vi "take img.vi"() -> ()   [LabVIEW 2019]
uses:
  <vilib>/userDefined/High Color/IMAQdx.ctl
  <vilib>/vision/driver/NI_Vision_Acquisition_Software.lvlib
panel:
  out "error out":errorcluster
  in  "stop":bool
  in  "Boolean":bool
  out "Image":T1(plugin-control)
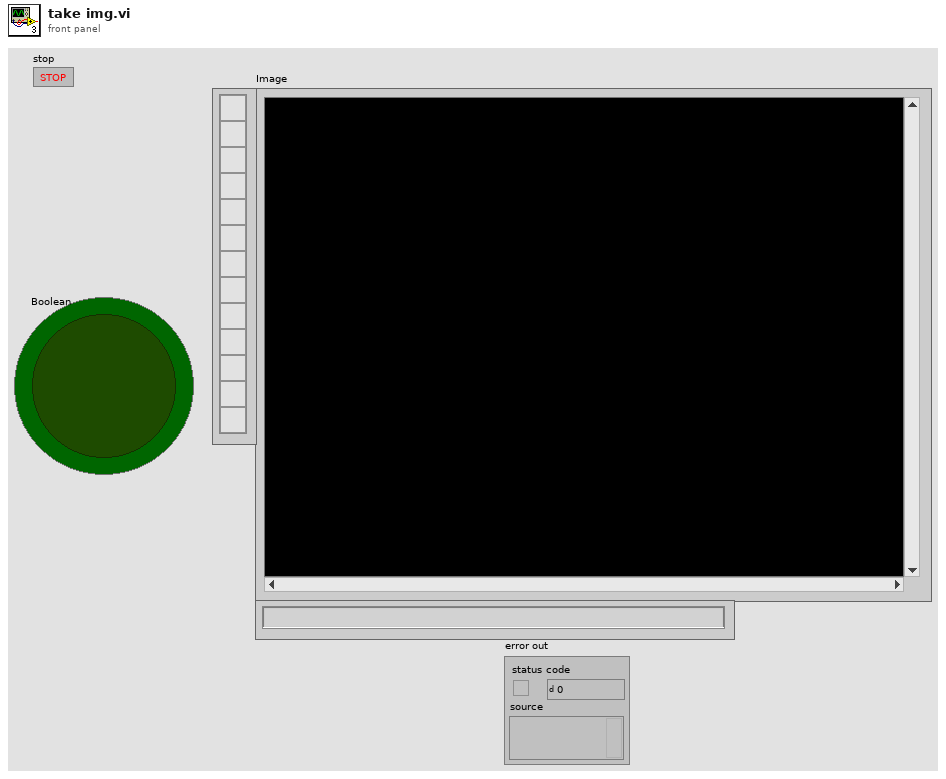
[diagram p1: front panel]
types:
  T1 = typedef "IMAQ Image.ctl" = refnum<image>
  T2 = typedef "IMAQdx.ctl" = refnum<k21>
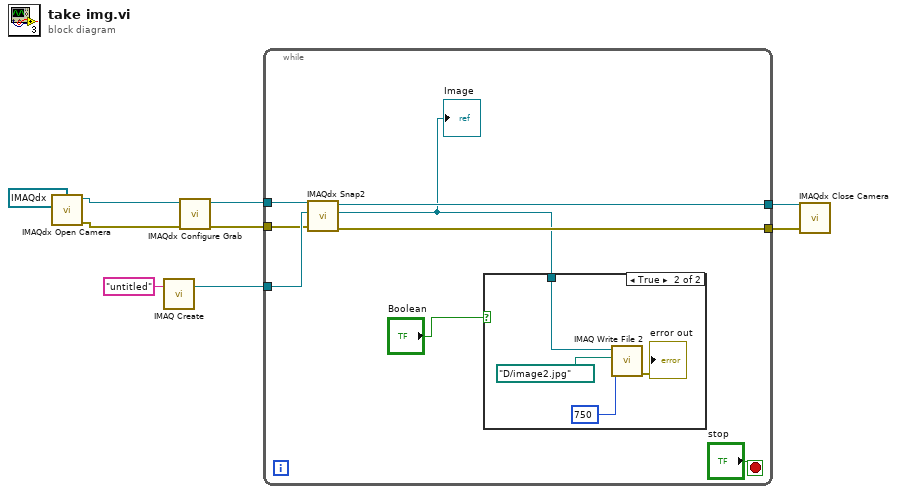
[diagram p0: block diagram]
diagram:
  n1 = call <vilib>:"IMAQdx Open Camera.vi"("Session In"=T2 "cam1") -> ("error out"=w2:errorcluster, "Session Out"=w8:T2)  [unwired: 9 in]
  n2 = call "IMAQ Create"("Image Name"="untitled") -> ("New Image"=w3:T1)  [unwired: 4 in, 1 out]
  n3 = call <vilib>:"IMAQdx Configure Grab.vi"("error in"=w2, "Session In"=w8) -> ("error out"=w1:errorcluster, "Session Out"=w7:T2)  [unwired: 8 in]
  n4 = while {
    tunnel: w7 -> [w17]
    tunnel: [w16] -> w6
    tunnel: [w15] -> w5
    tunnel: w3 -> [w14]
    tunnel: w1 -> [w13]
    stop <- "stop" stop-if-true
    n5 = call <vilib>:"IMAQdx Snap2.vi"("error in"=w13, "Image In"=w14, "Session In"=w17) -> ("error out"=w16:errorcluster, "Image Out"=w12:T1, "Session Out"=w15:T2)  [unwired: 6 in]
    "Image" <- w12
    n6 = case shown="True" "Boolean" {
      tunnel: w12 -> [_ w21]
      frame False {
      }
      frame True {
        n7 = call-poly "IMAQ Write File 2"("Image Quality"=u32 750, "File Path"=path "D:/image2.jpg", "Image"=w21) -> ("error out"=→"error out":errorcluster)  [unwired: 7 in, 1 out]
      }
    }
  }
  n8 = call <vilib>:"IMAQdx Close Camera.vi"("error in"=w6, "Session In"=w5) -> ()  [unwired: 9 in, 1 out]
